vi "Assign GPIO Pins.vi"(5 "EOT Pin (0: None)":i32(ring) items=["None", "EXT1", "EXT2", "EXT3", "EXT4", "EXT5", "EXT6", "EXT7"], 6 "SOT Pin (0: None)":i32(ring) items=["None", "EXT1", "EXT2", "EXT3", "EXT4", "EXT5", "EXT6", "EXT7"], 7 "Busy Pin (0: None)":i32(ring) items=["None", "EXT1", "EXT2", "EXT3", "EXT4", "EXT5", "EXT6", "EXT7"], 8 "error in (no error)":errorcluster, 9 "Result Pins":i32[](array[ring]) items=["EXT1"=1, "EXT2"=2, "EXT3"=3, "EXT4"=4, "EXT5"=5, "EXT6"=6, "EXT7"=7], 10 "Channel (1: Channel 1)":i32(ring)=1 items=["Channel 1"=1, "Channel 2"=2], 11 "VISA resource name":refnum<visa-resource-name>) -> (0 "error out":errorcluster, 3 "VISA resource name out":refnum<visa-resource-name>)   [LabVIEW 2012, in "Keysight B2980 Series.lvlib"]
doc: "Assigns the GPIO pins used for the result output and pin for specified signal line for the composite limit test."
uses:
  Keysight B2980 Series.lvlib
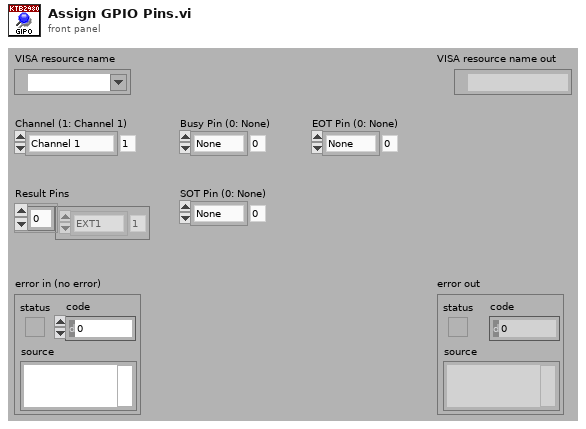
[diagram p1: front panel]
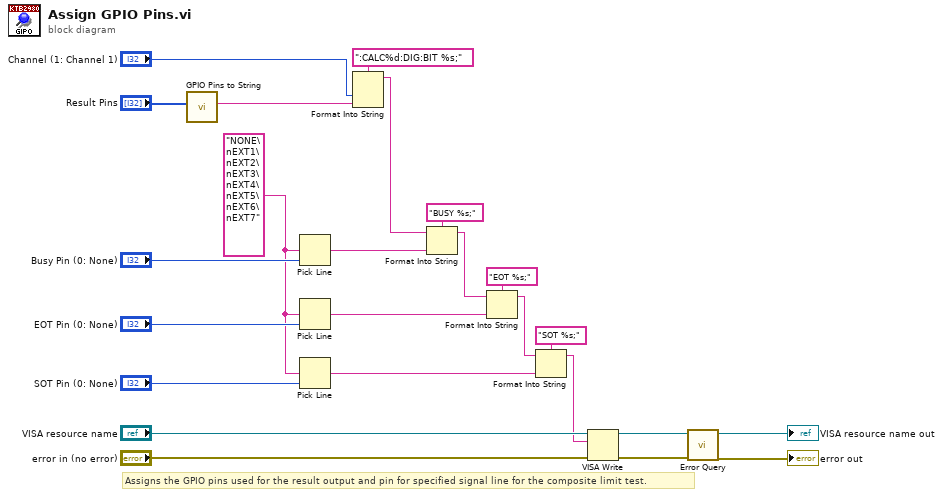
[diagram p0: block diagram]
diagram:
  w1 = "NONE\nEXT1\nEXT2\nEXT3\nEXT4\nEXT5\nEXT6\nEXT7"
  # "Assigns the GPIO pins used for the result output and pin for specified signal line for the composite limit test."
  n1 = call "GPIO Pins to String.vi"("Result Pins"="Result Pins") -> ("Result String"=w15:string)  [unwired: 10 out]
  n2 = Pick Line(multi-line string=w1, line index="Busy Pin (0: None)") -> (output string=w8:string)  [unwired: 1 out]
  n3 = Pick Line(multi-line string=w1, line index="EOT Pin (0: None)") -> (output string=w6:string)  [unwired: 1 out]
  n4 = Pick Line(multi-line string=w1, line index="SOT Pin (0: None)") -> (output string=w3:string)  [unwired: 1 out]
  n5 = Format Into String(format string=":CALC%d:DIG:BIT %s;", "Channel (1: Channel 1)", w15) -> (resulting string=w11:string)  [unwired: 2 in, 1 out]
  n6 = Format Into String(format string="BUSY %s;", initial string=w11, w8) -> (resulting string=w10:string)  [unwired: 1 in, 1 out]
  n7 = Format Into String(format string="EOT %s;", initial string=w10, w6) -> (resulting string=w9:string)  [unwired: 1 in, 1 out]
  n8 = Format Into String(format string="SOT %s;", initial string=w9, w3) -> (resulting string=w2:string)  [unwired: 1 in, 1 out]
  n9 = VISA Write(VISA resource name="VISA resource name", write buffer=w2, error in (no error)="error in (no error)") -> (VISA resource name out=w20:refnum<visa-resource-name>, error out=w19:errorcluster)  [unwired: 1 out]
  n10 = call "Error Query.vi"("error in (no error)"=w19, "VISA resource name"=w20) -> ("error out"=→"error out":errorcluster, "VISA resource name out"=→"VISA resource name out":refnum<visa-resource-name>)  [unwired: 8 out]
